vi "HCC Washer Cluster Arrays ReadWrite.vi"(0 "Array Label":string(combo)="Aisle1", 1 "Write?":bool, 5 "configuration file path":path=path "C:/data/Wilt Backup.ini", 7 "Array Washers In":T1[](array[typedef]) {"Cycle Count" format="%05d"}, 11 "error in (no error)":errorcluster) -> (8 "Array Washers Out":T1[](array[typedef]) {"Cycle Count" format="%05d"}, 15 "error out":errorcluster)   [LabVIEW 2009]
uses:
  <vilib>/Utility/VariantDataType/Type.ctl
  Washer.ctl
  Dryer Wilt/Dryer Details.ctl
  <vilib>/Utility/config.llb/Write Key (Double).vi
  <vilib>/Utility/config.llb/Write Key (String).vi
  <vilib>/Utility/config.llb/Write Key (Path).vi
  <vilib>/Utility/config.llb/Write Key (I32).vi
  <vilib>/Utility/config.llb/Write Key (U32).vi
  <vilib>/Utility/config.llb/Write Key (Boolean).vi
  <vilib>/Utility/config.llb/Read Key (String).vi
  <vilib>/Utility/config.llb/Read Key (Double).vi
  <vilib>/Utility/config.llb/Read Key (Path).vi
  <vilib>/Utility/config.llb/Read Key (I32).vi
  <vilib>/Utility/config.llb/Read Key (U32).vi
  <vilib>/Utility/config.llb/Read Key (Boolean).vi
  <vilib>/Utility/config.llb/NI_LVConfig.lvlib
  <vilib>/Utility/VariantDataType/VariantType.lvlib
panel:
  out "Local Control?":bool
  in  "Array Dryers Display":T1[](array[typedef]) {"Cycle Count" format="%05d"}
  out "value":string
  in  "Washer Variable":T1 {"Cycle Count" format="%05d"}
  out "Label.Text 2":string
  out "Type Enum 2":T3
  out "String array out":string="[1,23-2-3]\n[4-3,22-2]\n[3-4,01-8]\n[0-7-6,66]"
  out "Label.Text":string
  out "Type Enum":T3
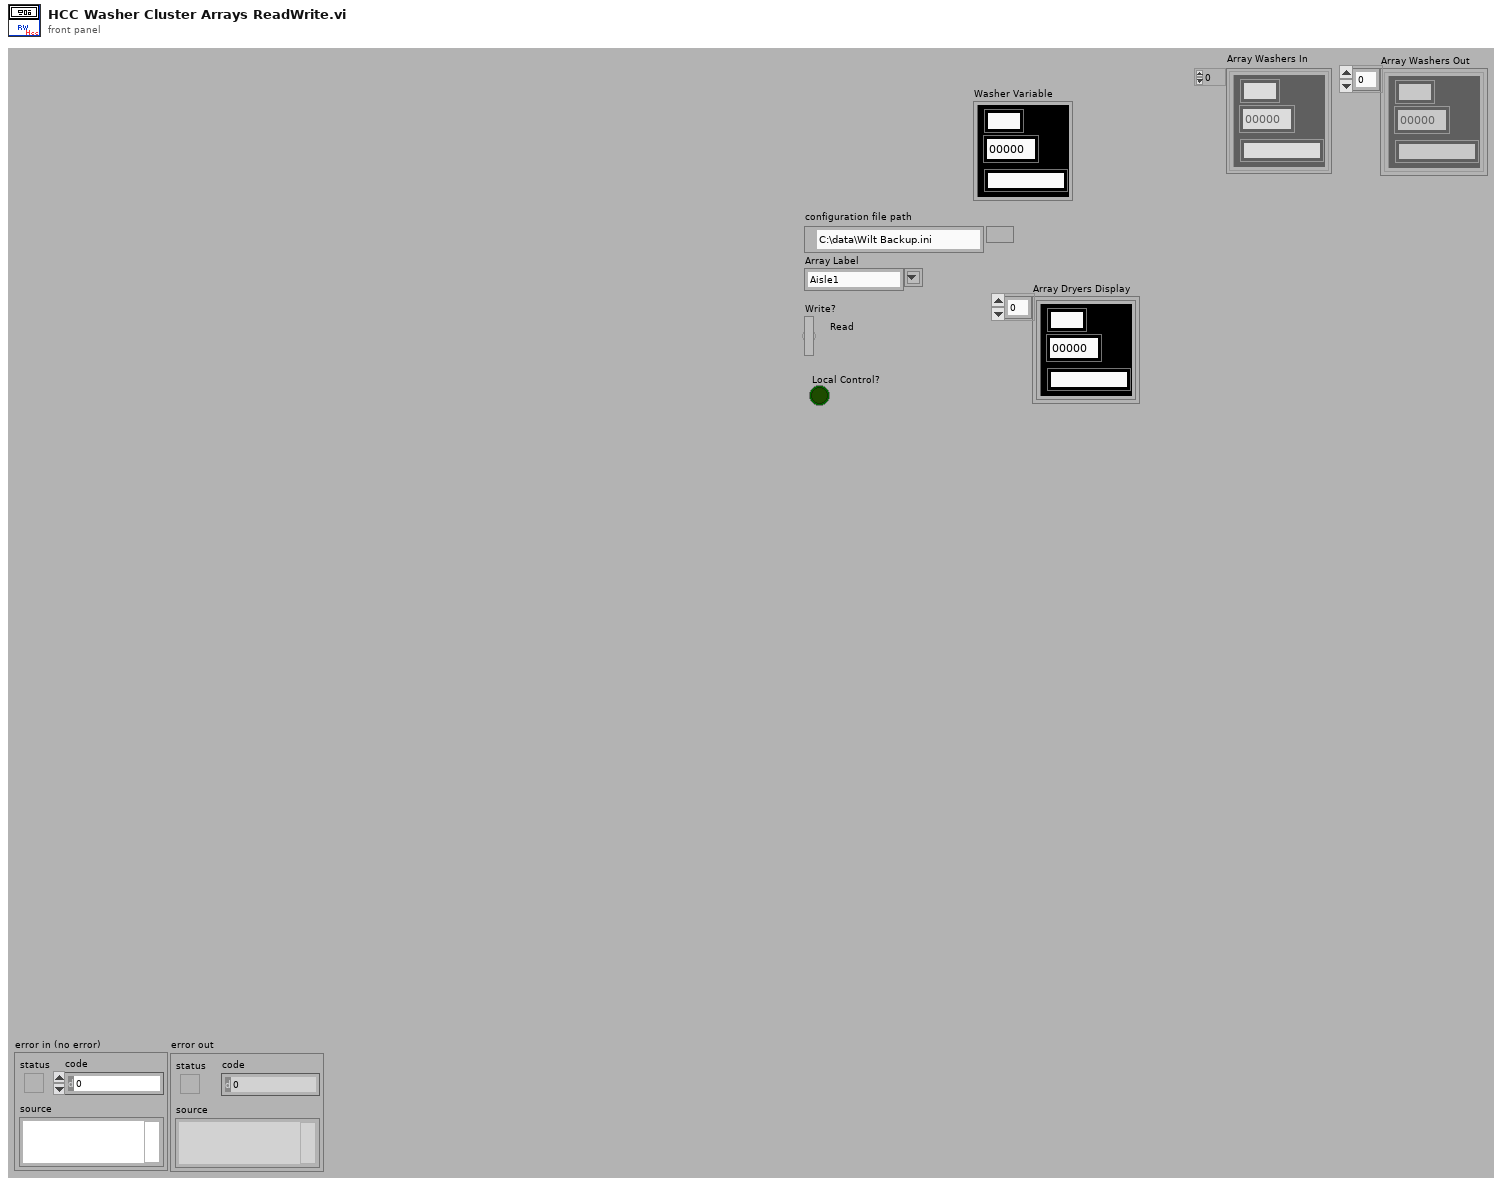
[diagram p1: front panel]
types:
  T1 = typedef "Washer.ctl" = cluster{"Serial Number":string, "Cycle Count":i32, "Station Number":string, "Dryer Details":T2, "Sample Record(t, CC, ASCII, Status ) ":string[], "Hist Record(Cycle Count, t-comp) ":string[][], "Status Color":u32, "Com Port":u8, "Bad Com Count":i32, "Boolean":bool}
  T2 = typedef "Dryer Details.ctl" = cluster{"Station":string, "Cycle Count":string, "Status":string, "Debug ASCII":string, "Notes":string, "File: Current Cycle":string, "Serial Number":string, "Total Time On":string, "TR Number":string, "File: Historic Data":string}
  T3 = typedef "VariantType.lvlib/Type.ctl" = enum8{"Invalid Type", "Void", "I8", "I16", "I32", "I64", "U8", "U16", "U32", "U64", "Single Float", "Double Float", "Extended Float", "Single Complex", "Double Complex", "Extended Complex", "Enum U8", "Enum U16", "Enum U32", "Enum U64", "Single Float With Unit", "Double Float With Unit", "Extended Float With Unit", "Single Complex with Unit", "Double Complex with Unit", "Extended Complex with Unit", "Boolean", "String", "Path", "Picture", "Tag", "Array", "Cluster", "Variant", "LV Variant", "Waveform", "Timestamp", "Digital Waveform", "Digital Data", "ExpressData", "Refnum", "External Data", "VI", "Poly VI", "LabVIEW Class Instance", "Fixed Point"}
  T4 = typedef "NI_LVConfig.lvlib/Config Data RefNum.ctl" = refnum<k1>
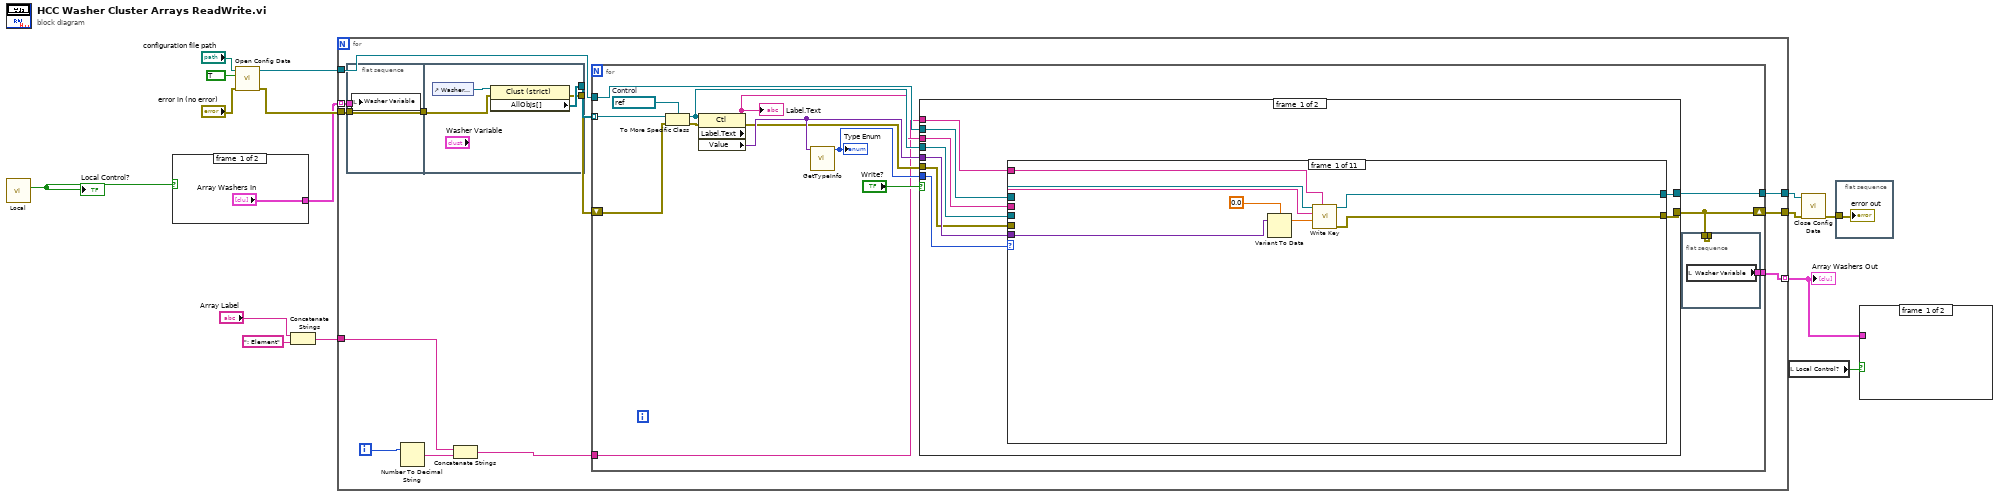
[diagram p0: block diagram]
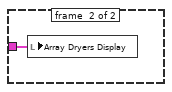
[diagram p2: hidden frame]
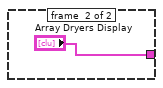
[diagram p3: hidden frame]
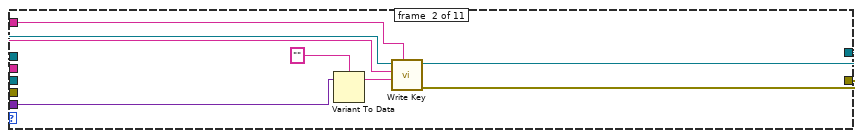
[diagram p4: hidden frame]
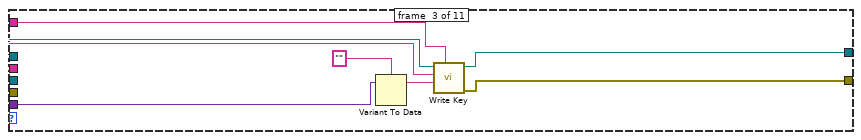
[diagram p5: hidden frame]
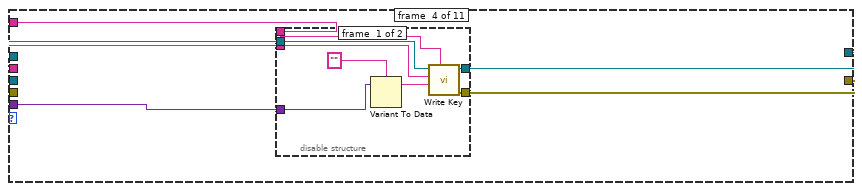
[diagram p6: hidden frame]
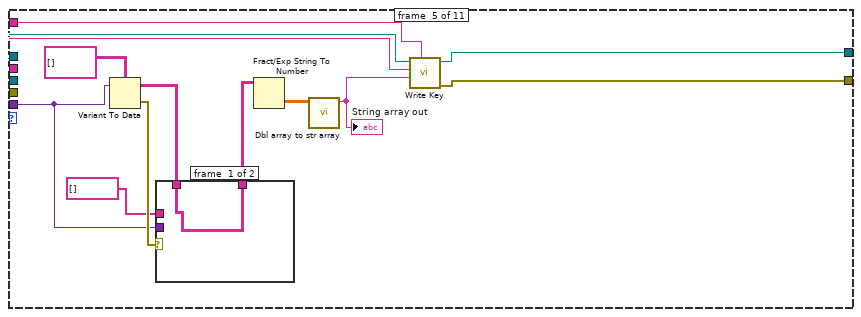
[diagram p8: hidden frame]
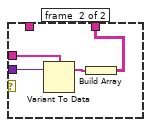
[diagram p9: hidden frame]
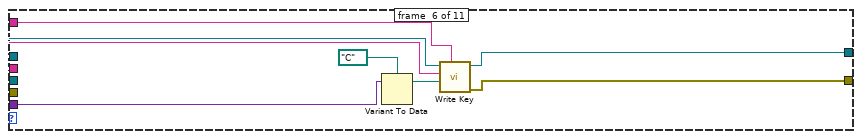
[diagram p10: hidden frame]
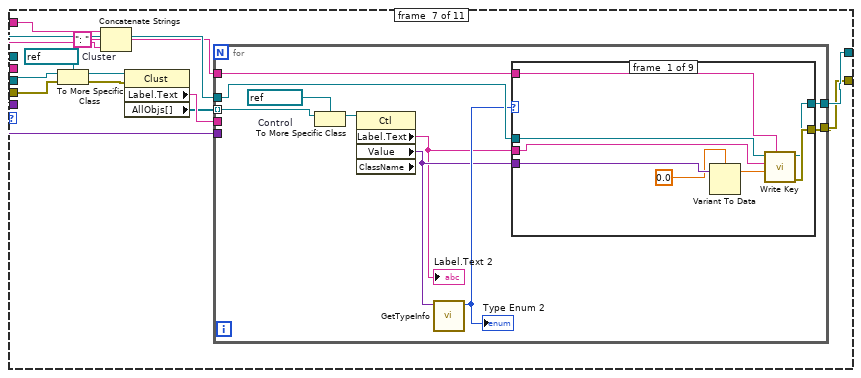
[diagram p11: hidden frame]
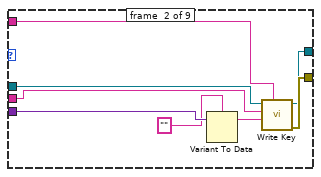
[diagram p12: hidden frame]
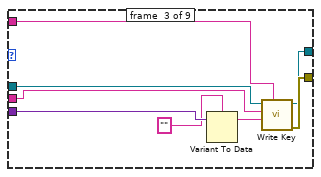
[diagram p13: hidden frame]
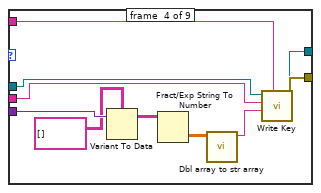
[diagram p14: hidden frame]
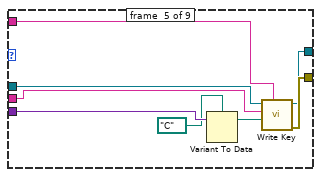
[diagram p15: hidden frame]
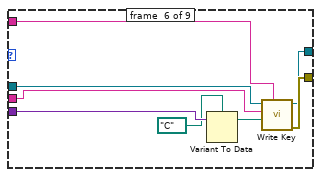
[diagram p16: hidden frame]
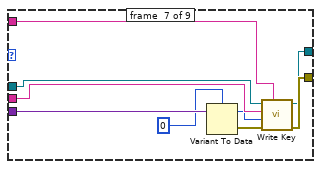
[diagram p17: hidden frame]
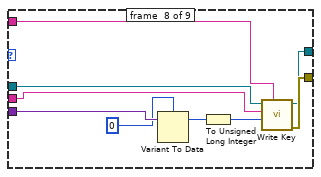
[diagram p18: hidden frame]
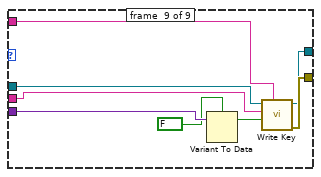
[diagram p19: hidden frame]
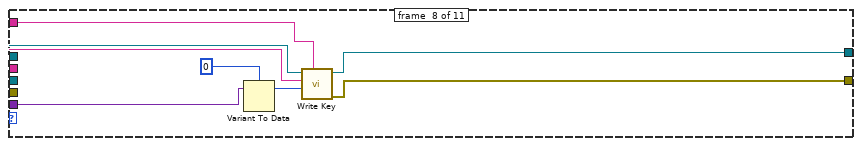
[diagram p20: hidden frame]
diagram:
  n1 = call "Local.vi"() -> ("Local?"=w1:bool)  [unwired: 11 in]
  "Local Control?" <- w1
  n2 = case shown="True" w1 {
    tunnel: ["Array Washers In" "Array Dryers Display"] -> w3
    frame #0 {
    }
    frame #1 {
    }
  }
  n3 = call <vilib>:"Open Config Data.vi"("error in (no error)"="error in (no error)", "create file if necessary (T)"=TRUE, "configuration file path"="configuration file path") -> ("error out"=w11:errorcluster, "refnum"=w13:T4)  [unwired: 6 in, 1 out]
  n4 = Concatenate Strings("Array Label", ": Element" ("string")) -> (w8:string)
  n5 = for {
    tunnel: w11 -> [w29]
    tunnel: w3 -> [w25] mode=indexing
    tunnel: w13 -> [w27]
    tunnel: w8 -> [w23]
    tunnel: [w20] -> w6
    tunnel: [w19] -> w5
    tunnel: [w18] -> w4 mode=indexing
    i -> [w21]
    n6 = flat-sequence {
      tunnel: w29 -> [w32]
      tunnel: [w32] -> w26
      tunnel: w25 -> [w31]
      tunnel: [w36] -> w30
      tunnel: [w34] -> w28
      tunnel: w26 -> [w35]
      frame #0 {
        n7 = local write "Washer Variable"(w31) -> ()
      }
      frame #1 {
        n8 = control-ref of="Washer Variable"() -> (w33:refnum<vi>)
        n9 = property class="Clust (strict)"(reference=w33, error in=w35) -> (error out=w34:errorcluster, "AllObjs[]"=w36:refnum<vi>[])  [unwired: 1 out]
      }
    }
    n10 = Number To Decimal String(number=w21) -> (decimal integer string=w24:string)  [unwired: 1 in]
    n11 = Concatenate Strings(w23, w24) -> (w22:string)
    n12 = for {
      tunnel: w30 -> [w51] mode=indexing
      tunnel: w27 -> [w49]
      tunnel: [w48] -> w19
      shift-right: [w38] -> w20
      shift-left: w28 -> [w47]
      tunnel: w22 -> [w39]
      tunnel: [w37] -> w18
      w50 = refnum<vi> refnum  # Control
      n13 = To More Specific Class(target class=w50, reference=w51, error in=w47) -> (specific class reference=w41:refnum<vi>, error out=w42:errorcluster)
      n14 = property class="Ctl"(reference=w41, error in=w42) -> (error out=w43:errorcluster, "Label.Text"=w40:string, "Value"=w44:variant)  [unwired: 1 out]
      "Label.Text" <- w40
      n15 = call <vilib>:"GetTypeInfo.vi"("Variant"=w44) -> ("Type Enum"=w45:T3)  [unwired: 6 in, 4 out]
      "Type Enum" <- w45
      n16 = case shown="False" "Write?" {
        tunnel: w39 -> [w62 w269]
        tunnel: w40 -> [w61 w268]
        tunnel: w44 -> [w60 w261]
        tunnel: w49 -> [w59 w267]
        tunnel: [w58 w266] -> w38
        tunnel: [w57 w265] -> w48
        tunnel: w41 -> [w54 w264]
        tunnel: w45 -> [w56 w263]
        tunnel: w43 -> [w55 w262]
        frame #0 {
          n17 = case shown="\"Array\"" w56 {
            tunnel: w62 -> [w70 w78 w86 w92 w113 w126 w129 w235 w243 w252 w260]
            tunnel: w61 -> [w69 w77 w85 w91 w112 w125 w128 w234 w242 w251 w259]
            tunnel: w60 -> [w68 w76 w84 w90 w102 w124 w137 w233 w241 w250 w258]
            tunnel: w59 -> [w67 w75 w83 w89 w111 w123 w131 w232 w240 w249 w257]
            tunnel: [w66 w74 w82 w88 w110 w122 w135 w231 w239 w248 w256] -> w58
            tunnel: [w65 w73 w81 w87 w109 w121 w136 w230 w238 w247 w255] -> w57
            tunnel: w55 -> [_ _ _ _ _ _ w138 _ _ _ _]
            tunnel: w54 -> [_ _ _ _ _ _ w133 _ _ _ _]
            frame #0 {
              n18 = Variant To Data(Variant=w68, type=0.0) -> (data=w64:dbl)  [unwired: 1 in, 1 out]
              n19 = call-poly <vilib>:"Write Key.vi"("section"=w70, "value"=w64, "key"=w69, "refnum"=w67) -> ("error out"=w66:errorcluster, "refnum out"=w65:T4)  [unwired: 5 in, 1 out]
            }
            frame #1 {
              n20 = Variant To Data(Variant=w76, type="" ("Label.Text")) -> (data=w72:string)  [unwired: 1 in, 1 out]
              n21 = call-poly <vilib>:"Write Key.vi"("section"=w78, "value"=w72, "key"=w77, "refnum"=w75) -> ("error out"=w74:errorcluster, "refnum out"=w73:T4)  [unwired: 5 in, 1 out]
            }
            frame #2 {
              n22 = Variant To Data(Variant=w84, type="" ("Label.Text")) -> (data=w80:string)  [unwired: 1 in, 1 out]
              n23 = call-poly <vilib>:"Write Key.vi"("section"=w86, "value"=w80, "key"=w85, "refnum"=w83) -> ("error out"=w82:errorcluster, "refnum out"=w81:T4)  [unwired: 5 in, 1 out]
            }
            frame #3 {
              n24 = disable-structure shown="Enabled" {
                disable-tunnel: w92 -> [w100 _]
                disable-tunnel: w91 -> [w99 _]
                disable-tunnel: w90 -> [w98 _]
                disable-tunnel: w89 -> [w97 _]
                disable-tunnel: [w96 _] -> w88
                disable-tunnel: [w95 _] -> w87
                frame #0 {
                  n25 = Variant To Data(Variant=w98, type="" ("Label.Text")) -> (data=w94:string)  [unwired: 1 in, 1 out]
                  n26 = call-poly <vilib>:"Write Key.vi"("section"=w100, "value"=w94, "key"=w99, "refnum"=w97) -> ("error out"=w96:errorcluster, "refnum out"=w95:T4)  [unwired: 5 in, 1 out]
                }
                frame #1 {
                }
              }
            }
            frame #4 {
              n27 = Variant To Data(Variant=w102, type=string[][] []) -> (error out=w105:errorcluster, data=w104:string[][])  [unwired: 1 in]
              n28 = case shown="Error" w105 {
                tunnel: [w114 w115] -> w103
                tunnel: w104 -> [w114 _]
                tunnel: w102 -> [_ w118]
                tunnel: string[] [] -> [_ w117]
                frame #0 {
                }
                frame #1 {
                  n29 = Variant To Data(Variant=w118, type=w117) -> (data=w116:string[])  [unwired: 1 in, 1 out]
                  n30 = Build Array(w116) -> (w115:string[][])
                }
              }
              n31 = Fract/Exp String To Number(string=w103) -> (number=w107:dbl[][])  [unwired: 3 in, 1 out]
              n32 = call "Dbl array to str array.vi"("Array in"=w107) -> ("String array out"=w106:string)  [unwired: 9 in, 1 out]
              "String array out" <- w106
              n33 = call-poly <vilib>:"Write Key.vi"("section"=w113, "value"=w106, "key"=w112, "refnum"=w111) -> ("error out"=w110:errorcluster, "refnum out"=w109:T4)  [unwired: 5 in, 1 out]
            }
            frame #5 {
              n34 = Variant To Data(Variant=w124, type=path "C:/" ("configuration file path 2")) -> (data=w120:path)  [unwired: 1 in, 1 out]
              n35 = call-poly <vilib>:"Write Key.vi"("section"=w126, "value"=w120, "key"=w125, "refnum"=w123) -> ("error out"=w122:errorcluster, "refnum out"=w121:T4)  [unwired: 5 in, 1 out]
            }
            frame #6 {
              w141 = refnum<vi> refnum  # Cluster
              n36 = To More Specific Class(target class=w141, reference=w133, error in=w138) -> (specific class reference=w140:refnum<vi>, error out=w139:errorcluster)
              n37 = Concatenate Strings(w129, ": " ("string"), w128) -> (w130:string)
              n38 = property class="Clust"(reference=w140, error in=w139) -> ("Label.Text"=w134:string, "AllObjs[]"=w132:refnum<vi>[])  [unwired: 2 out]
              n39 = for {
                tunnel: w137 -> [_]
                tunnel: w130 -> [w151]
                tunnel: w132 -> [w146] mode=indexing
                tunnel: [w150] -> w136
                tunnel: [w149] -> w135
                tunnel: w134 -> [_]
                tunnel: w131 -> [w145]
                w148 = refnum<vi> refnum  # Control
                n40 = To More Specific Class(target class=w148, reference=w146) -> (specific class reference=w147:refnum<vi>)  [unwired: 1 in, 1 out]
                n41 = property class="Ctl" props=["Label", "Text", "Value", "ClassName"](reference=w147) -> ("Label.Text"=w142:string, "Value"=w143:variant)  [unwired: 1 in, 3 out]
                "Label.Text 2" <- w142
                n42 = call <vilib>:"GetTypeInfo.vi"("Variant"=w143) -> ("Type Enum"=w144:T3)  [unwired: 6 in, 4 out]
                "Type Enum 2" <- w144
                n43 = case shown="\"Array\"" w144 {
                  tunnel: w151 -> [w159 w167 w175 w185 w187 w201 w210 w219 w227]
                  tunnel: w142 -> [w158 w166 w168 w184 w186 w200 w209 w218 w226]
                  tunnel: w143 -> [w157 w165 w174 w183 w193 w199 w208 w217 w225]
                  tunnel: w145 -> [w152 w160 w169 w176 w188 w194 w202 w211 w220]
                  tunnel: [w156 w164 w173 w182 w192 w198 w207 w216 w224] -> w149
                  tunnel: [w155 w163 w172 w181 w191 w197 w206 w215 w223] -> w150
                  frame #0 {
                    n44 = Variant To Data(Variant=w157, type=0.0) -> (data=w153:dbl)  [unwired: 1 in, 1 out]
                    n45 = call-poly <vilib>:"Write Key.vi"("section"=w159, "value"=w153, "key"=w158, "refnum"=w152) -> ("error out"=w156:errorcluster, "refnum out"=w155:T4)  [unwired: 5 in, 1 out]
                  }
                  frame #1 {
                    n46 = Variant To Data(Variant=w165, type="" ("Label.Text")) -> (data=w161:string)  [unwired: 1 in, 1 out]
                    n47 = call-poly <vilib>:"Write Key.vi"("section"=w167, "value"=w161, "key"=w166, "refnum"=w160) -> ("error out"=w164:errorcluster, "refnum out"=w163:T4)  [unwired: 5 in, 1 out]
                  }
                  frame #2 {
                    n48 = Variant To Data(Variant=w174, type="" ("Label.Text")) -> (data=w170:string)  [unwired: 1 in, 1 out]
                    n49 = call-poly <vilib>:"Write Key.vi"("section"=w175, "value"=w170, "key"=w168, "refnum"=w169) -> ("error out"=w173:errorcluster, "refnum out"=w172:T4)  [unwired: 5 in, 1 out]
                  }
                  frame #3 {
                    n50 = Variant To Data(Variant=w183, type=string[][] []) -> (data=w179:string[][])  [unwired: 1 in, 1 out]
                    n51 = Fract/Exp String To Number(string=w179) -> (number=w178:dbl[][])  [unwired: 3 in, 1 out]
                    n52 = call "Dbl array to str array.vi"("Array in"=w178) -> ("String array out"=w177:string)  [unwired: 9 in, 1 out]
                    n53 = call-poly <vilib>:"Write Key.vi"("section"=w185, "value"=w177, "key"=w184, "refnum"=w176) -> ("error out"=w182:errorcluster, "refnum out"=w181:T4)  [unwired: 5 in, 1 out]
                  }
                  frame #4 {
                    n54 = Variant To Data(Variant=w193, type=path "C:/" ("configuration file path 2")) -> (data=w189:path)  [unwired: 1 in, 1 out]
                    n55 = call-poly <vilib>:"Write Key.vi"("section"=w187, "value"=w189, "key"=w186, "refnum"=w188) -> ("error out"=w192:errorcluster, "refnum out"=w191:T4)  [unwired: 5 in, 1 out]
                  }
                  frame #5 {
                    n56 = Variant To Data(Variant=w199, type=path "C:/" ("configuration file path 2")) -> (data=w195:path)  [unwired: 1 in, 1 out]
                    n57 = call-poly <vilib>:"Write Key.vi"("section"=w201, "value"=w195, "key"=w200, "refnum"=w194) -> ("error out"=w198:errorcluster, "refnum out"=w197:T4)  [unwired: 5 in, 1 out]
                  }
                  frame #6 {
                    n58 = Variant To Data(Variant=w208, type=0) -> (error out=w204:errorcluster, data=w203:i32)  [unwired: 1 in]
                    n59 = call-poly <vilib>:"Write Key.vi"("section"=w210, "error in (no error)"=w204, "value"=w203, "key"=w209, "refnum"=w202) -> ("error out"=w207:errorcluster, "refnum out"=w206:T4)  [unwired: 4 in, 1 out]
                  }
                  frame #7 {
                    n60 = Variant To Data(Variant=w217, type=u8 0) -> (data=w214:u8)  [unwired: 1 in, 1 out]
                    n61 = To Unsigned Long Integer(number=w214) -> (unsigned 32bit integer=w212:u32)
                    n62 = call-poly <vilib>:"Write Key.vi"("section"=w219, "value"=w212, "key"=w218, "refnum"=w211) -> ("error out"=w216:errorcluster, "refnum out"=w215:T4)  [unwired: 5 in, 1 out]
                  }
                  frame #8 {
                    n63 = Variant To Data(Variant=w225, type=FALSE ("Write? 2")) -> (data=w222:bool)  [unwired: 1 in, 1 out]
                    n64 = call-poly <vilib>:"Write Key.vi"("section"=w227, "value"=w222, "key"=w226, "refnum"=w220) -> ("error out"=w224:errorcluster, "refnum out"=w223:T4)  [unwired: 5 in, 1 out]
                  }
                }
              }
            }
            frame #7 {
              n65 = Variant To Data(Variant=w233, type=0) -> (data=w229:i32)  [unwired: 1 in, 1 out]
              n66 = call-poly <vilib>:"Write Key.vi"("section"=w235, "value"=w229, "key"=w234, "refnum"=w232) -> ("error out"=w231:errorcluster, "refnum out"=w230:T4)  [unwired: 5 in, 1 out]
            }
            frame #8 {
              n67 = Variant To Data(Variant=w241, type=0) -> (data=w237:i32)  [unwired: 1 in, 1 out]
              n68 = call-poly <vilib>:"Write Key.vi"("section"=w243, "value"=w237, "key"=w242, "refnum"=w240) -> ("error out"=w239:errorcluster, "refnum out"=w238:T4)  [unwired: 5 in, 1 out]
            }
            frame #9 {
              n69 = Variant To Data(Variant=w250, type=u8 0) -> (data=w246:u8)  [unwired: 1 in, 1 out]
              n70 = To Unsigned Long Integer(number=w246) -> (unsigned 32bit integer=w244:u32)
              n71 = call-poly <vilib>:"Write Key.vi"("section"=w252, "value"=w244, "key"=w251, "refnum"=w249) -> ("error out"=w248:errorcluster, "refnum out"=w247:T4)  [unwired: 5 in, 1 out]
            }
            frame #10 {
              n72 = Variant To Data(Variant=w258, type=FALSE ("Write? 2")) -> (data=w254:bool)  [unwired: 1 in, 1 out]
              n73 = call-poly <vilib>:"Write Key.vi"("section"=w260, "value"=w254, "key"=w259, "refnum"=w257) -> ("error out"=w256:errorcluster, "refnum out"=w255:T4)  [unwired: 5 in, 1 out]
            }
          }
        }
        frame #1 {
          n74 = case shown="Default" w263 {
            tunnel: w269 -> [w277 w285 w293 w304 w312 w328 w421 w429 w437 w445 w453]
            tunnel: w268 -> [w276 w284 w292 w303 w319 w324 w428 w436 w444 w452 w460]
            tunnel: w267 -> [w275 w283 w291 w302 w318 w323 w427 w435 w443 w451 w459]
            tunnel: [w274 w282 w290 w301 w317 w321 w426 w434 w442 w450 w458] -> w266
            tunnel: [w273 w281 w289 w300 w316 w322 w425 w433 w441 w449 w457] -> w265
            tunnel: w264 -> [w271 w279 w287 w295 w314 w325 w423 w431 w439 w447 w455]
            tunnel: w262 -> [w270 w278 w286 w299 w313 w326 w422 w430 w438 w446 w454]
            tunnel: w261 -> [_ _ _ _ _ w327 _ _ _ _ _]
            frame #0 {
              n75 = call-poly <vilib>:"Read Key.vi"("section"=w277, "error in (no error)"=w270, "key"=w276, "refnum"=w275) -> ("error out"=w274:errorcluster, "value"=w272:string, "refnum out"=w273:T4)  [unwired: 4 in, 1 out]
              n76 = property class="Ctl"(reference=w271, "Value"=w272) -> ()  [unwired: 1 in, 2 out]
            }
            frame #1 {
              n77 = call-poly <vilib>:"Read Key.vi"("section"=w285, "error in (no error)"=w278, "key"=w284, "refnum"=w283) -> ("error out"=w282:errorcluster, "value"=w280:dbl, "refnum out"=w281:T4)  [unwired: 4 in, 1 out]
              n78 = property class="Ctl"(reference=w279, "Value"=w280) -> ()  [unwired: 1 in, 2 out]
            }
            frame #2 {
              n79 = call-poly <vilib>:"Read Key.vi"("section"=w293, "error in (no error)"=w286, "key"=w292, "refnum"=w291) -> ("error out"=w290:errorcluster, "value"=w288:string, "refnum out"=w289:T4)  [unwired: 4 in, 1 out]
              n80 = property class="Ctl"(reference=w287, "Value"=w288) -> ()  [unwired: 1 in, 2 out]
            }
            frame #3 {
              n81 = call-poly <vilib>:"Read Key.vi"("section"=w304, "error in (no error)"=w299, "key"=w303, "refnum"=w302) -> ("error out"=w301:errorcluster, "value"=w298:string, "refnum out"=w300:T4)  [unwired: 4 in, 1 out]
              "value" <- w298
              n82 = call "Str array to dbl array.vi"("String array in"=w298) -> ("Double array out"=w297:dbl[][])  [unwired: 9 in, 1 out]
              n83 = Number To Fractional String(number=w297) -> (F-format string=w294:string[][])  [unwired: 3 in]
              n84 = property class="Ctl"(reference=w295, "Value"=w294) -> (error out=w296:errorcluster)  [unwired: 1 in, 1 out]
              n85 = case shown="Error" w296 {
                tunnel: w295 -> [_ w311]
                tunnel: w294 -> [_ w310]
                frame #0 {
                }
                frame #1 {
                  n86 = Array Subset(array=w310, index (row)=0 ("index")) -> (w307:string[][])  [unwired: 3 in]
                  n87 = Array Size(array=w307) -> (size(s)=w306:i32[])
                  n88 = Multiply Array Elements(1:w306) -> (0:w305:i32)
                  n89 = Reshape Array(w307, w305) -> (w308:string[])
                  n90 = property class="Ctl"(reference=w311, "Value"=w308) -> ()  [unwired: 1 in, 2 out]
                }
              }
            }
            frame #4 {
              n91 = call-poly <vilib>:"Read Key.vi"("section"=w312, "error in (no error)"=w313, "key"=w319, "refnum"=w318) -> ("error out"=w317:errorcluster, "value"=w315:path, "refnum out"=w316:T4)  [unwired: 4 in, 1 out]
              n92 = property class="Ctl"(reference=w314, "Value"=w315) -> ()  [unwired: 1 in, 2 out]
            }
            frame #5 {
              w335 = refnum<vi> refnum  # Cluster
              n93 = To More Specific Class(target class=w335, reference=w325, error in=w326) -> (specific class reference=w334:refnum<vi>, error out=w333:errorcluster)
              n94 = Concatenate Strings(w328, ": " ("string"), w324) -> (w330:string)
              n95 = property class="Clust"(reference=w334, error in=w333) -> (error out=w320:errorcluster, "Label.Text"=w332:string, "AllObjs[]"=w331:refnum<vi>[])  [unwired: 1 out]
              n96 = for {
                tunnel: w327 -> [_]
                tunnel: w330 -> [w338]
                tunnel: w331 -> [w345] mode=indexing
                tunnel: [w337] -> w322
                tunnel: [w341] -> w321
                tunnel: w332 -> [_]
                tunnel: w323 -> [w340]
                tunnel: w320 -> [w342]
                w347 = refnum<vi> refnum  # Control
                n97 = To More Specific Class(target class=w347, reference=w345) -> (specific class reference=w346:refnum<vi>)  [unwired: 1 in, 1 out]
                n98 = property class="Ctl"(reference=w346) -> (reference out=w339:refnum<vi>, "Label.Text"=w343:string, "Value"=w344:variant)  [unwired: 1 in, 1 out]
                n99 = call <vilib>:"GetTypeInfo.vi"("Variant"=w344) -> ("Type Enum"=w336:T3)  [unwired: 6 in, 4 out]
                n100 = case shown="\"Array\"" w336 {
                  tunnel: w338 -> [w355 w363 w371 w380 w381 w389 w397 w405 w413]
                  tunnel: w343 -> [w354 w362 w370 w379 w388 w396 w404 w412 w420]
                  tunnel: w340 -> [w353 w361 w369 w378 w387 w395 w403 w411 w419]
                  tunnel: [w352 w360 w368 w377 w386 w394 w402 w410 w418] -> w341
                  tunnel: [w351 w359 w367 w376 w385 w393 w401 w409 w417] -> w337
                  tunnel: w339 -> [w349 w357 w365 w375 w383 w391 w399 w407 w415]
                  tunnel: w342 -> [w348 w356 w364 w374 w382 w390 w398 w406 w414]
                  frame #0 {
                    n101 = call-poly <vilib>:"Read Key.vi"("section"=w355, "error in (no error)"=w348, "key"=w354, "refnum"=w353) -> ("error out"=w352:errorcluster, "value"=w350:string, "refnum out"=w351:T4)  [unwired: 4 in, 1 out]
                    n102 = property class="Ctl"(reference=w349, "Value"=w350) -> ()  [unwired: 1 in, 2 out]
                  }
                  frame #1 {
                    n103 = call-poly <vilib>:"Read Key.vi"("section"=w363, "error in (no error)"=w356, "key"=w362, "refnum"=w361) -> ("error out"=w360:errorcluster, "value"=w358:dbl, "refnum out"=w359:T4)  [unwired: 4 in, 1 out]
                    n104 = property class="Ctl"(reference=w357, "Value"=w358) -> ()  [unwired: 1 in, 2 out]
                  }
                  frame #2 {
                    n105 = call-poly <vilib>:"Read Key.vi"("section"=w371, "error in (no error)"=w364, "key"=w370, "refnum"=w369) -> ("error out"=w368:errorcluster, "value"=w366:string, "refnum out"=w367:T4)  [unwired: 4 in, 1 out]
                    n106 = property class="Ctl"(reference=w365, "Value"=w366) -> ()  [unwired: 1 in, 2 out]
                  }
                  frame #3 {
                    n107 = call-poly <vilib>:"Read Key.vi"("section"=w380, "error in (no error)"=w374, "key"=w379, "refnum"=w378) -> ("error out"=w377:errorcluster, "value"=w373:string, "refnum out"=w376:T4)  [unwired: 4 in, 1 out]
                    n108 = call "Str array to dbl array.vi"("String array in"=w373) -> ("Double array out"=w372:dbl[][])  [unwired: 9 in, 1 out]
                    n109 = property class="Ctl"(reference=w375, "Value"=w372) -> ()  [unwired: 1 in, 2 out]
                  }
                  frame #4 {
                    n110 = call-poly <vilib>:"Read Key.vi"("section"=w381, "error in (no error)"=w382, "key"=w388, "refnum"=w387) -> ("error out"=w386:errorcluster, "value"=w384:path, "refnum out"=w385:T4)  [unwired: 4 in, 1 out]
                    n111 = property class="Ctl"(reference=w383, "Value"=w384) -> ()  [unwired: 1 in, 2 out]
                  }
                  frame #5 {
                    n112 = call-poly <vilib>:"Read Key.vi"("section"=w389, "error in (no error)"=w390, "key"=w396, "refnum"=w395) -> ("error out"=w394:errorcluster, "value"=w392:i32, "refnum out"=w393:T4)  [unwired: 4 in, 1 out]
                    n113 = property class="Ctl"(reference=w391, "Value"=w392) -> ()  [unwired: 1 in, 2 out]
                  }
                  frame #6 {
                    n114 = call-poly <vilib>:"Read Key.vi"("section"=w397, "error in (no error)"=w398, "key"=w404, "refnum"=w403) -> ("error out"=w402:errorcluster, "value"=w400:u32, "refnum out"=w401:T4)  [unwired: 4 in, 1 out]
                    n115 = property class="Ctl"(reference=w399, "Value"=w400) -> ()  [unwired: 1 in, 2 out]
                  }
                  frame #7 {
                    n116 = call-poly <vilib>:"Read Key.vi"("section"=w405, "error in (no error)"=w406, "key"=w412, "refnum"=w411) -> ("error out"=w410:errorcluster, "value"=w408:bool, "refnum out"=w409:T4)  [unwired: 4 in, 1 out]
                    n117 = property class="Ctl"(reference=w407, "Value"=w408) -> ()  [unwired: 1 in, 2 out]
                  }
                  frame #8 {
                    n118 = call-poly <vilib>:"Read Key.vi"("section"=w413, "error in (no error)"=w414, "key"=w420, "refnum"=w419) -> ("error out"=w418:errorcluster, "value"=w416:bool, "refnum out"=w417:T4)  [unwired: 4 in, 1 out]
                    n119 = property class="Ctl"(reference=w415, "Value"=w416) -> ()  [unwired: 1 in, 2 out]
                  }
                }
              }
            }
            frame #6 {
              n120 = call-poly <vilib>:"Read Key.vi"("section"=w421, "error in (no error)"=w422, "key"=w428, "refnum"=w427) -> ("error out"=w426:errorcluster, "value"=w424:i32, "refnum out"=w425:T4)  [unwired: 4 in, 1 out]
              n121 = property class="Ctl"(reference=w423, "Value"=w424) -> ()  [unwired: 1 in, 2 out]
            }
            frame #7 {
              n122 = call-poly <vilib>:"Read Key.vi"("section"=w429, "error in (no error)"=w430, "key"=w436, "refnum"=w435) -> ("error out"=w434:errorcluster, "value"=w432:u32, "refnum out"=w433:T4)  [unwired: 4 in, 1 out]
              n123 = property class="Ctl"(reference=w431, "Value"=w432) -> ()  [unwired: 1 in, 2 out]
            }
            frame #8 {
              n124 = call-poly <vilib>:"Read Key.vi"("section"=w437, "error in (no error)"=w438, "key"=w444, "refnum"=w443) -> ("error out"=w442:errorcluster, "value"=w440:u32, "refnum out"=w441:T4)  [unwired: 4 in, 1 out]
              n125 = property class="Ctl"(reference=w439, "Value"=w440) -> ()  [unwired: 1 in, 2 out]
            }
            frame #9 {
              n126 = call-poly <vilib>:"Read Key.vi"("section"=w445, "error in (no error)"=w446, "key"=w452, "refnum"=w451) -> ("error out"=w450:errorcluster, "value"=w448:string, "refnum out"=w449:T4)  [unwired: 4 in, 1 out]
              n127 = property class="Ctl"(reference=w447, "Value"=w448) -> ()  [unwired: 1 in, 2 out]
            }
            frame #10 {
              n128 = call-poly <vilib>:"Read Key.vi"("section"=w453, "error in (no error)"=w454, "key"=w460, "refnum"=w459) -> ("error out"=w458:errorcluster, "value"=w456:bool, "refnum out"=w457:T4)  [unwired: 4 in, 1 out]
              n129 = property class="Ctl"(reference=w455, "Value"=w456) -> ()  [unwired: 1 in, 2 out]
            }
          }
        }
      }
      n130 = flat-sequence {
        tunnel: [w53] -> _
        tunnel: w38 -> [w53]
        tunnel: [w52] -> w37
        frame #0 {
          n131 = local read "Washer Variable"() -> (w52:T1)
        }
      }
    }
  }
  "Array Washers Out" <- w4
  n132 = local read "Local Control?"() -> (w2:bool)
  n133 = call <vilib>:"Close Config Data.vi"("error in (no error)"=w6, "refnum"=w5) -> ("error out"=w7:errorcluster)  [unwired: 8 in, 1 out]
  n134 = flat-sequence {
    tunnel: w7 -> [w461]
    frame #0 {
      "error out" <- w461
    }
  }
  n135 = case shown="True" w2 {
    tunnel: w4 -> [_ w462]
    frame #0 {
    }
    frame #1 {
      n136 = local write "Array Dryers Display"(w462) -> ()
    }
  }
